vi "SMO.UI.Splash.GetProtectedEvents.vi"(8 "error in (no error)":errorcluster, 11 "SMO.UI.Splash in":refnum<class "SMO.UI.Splash.lvclass">) -> (0 "error out":errorcluster, 2 "Protected Events":T1, 3 "SMO.UI.Splash out":refnum<class "SMO.UI.Splash.lvclass">)   [LabVIEW 2013, in "SMO.UI.Splash.lvclass"]
uses:
  SMO.UI.Splash.lvclass
  Typedefs/ProtectedEvents--Cluster.ctl
  Typedefs/DisplayMessage--Cluster.ctl
  SMO.UI.Splash.lvclass/SMO.UI.Splash.ctl
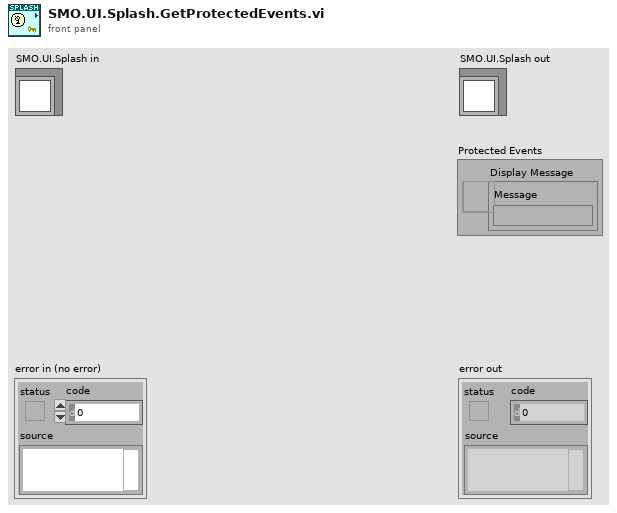
[diagram p1: front panel]
types:
  T1 = typedef "SMO.UI.Splash.lvclass/ProtectedEvents--Cluster.ctl" = cluster{"Display Message":T2}
  T2 = typedef "SMO.UI.Splash.lvclass/DisplayMessage--Cluster.ctl" = refnum<user-event>
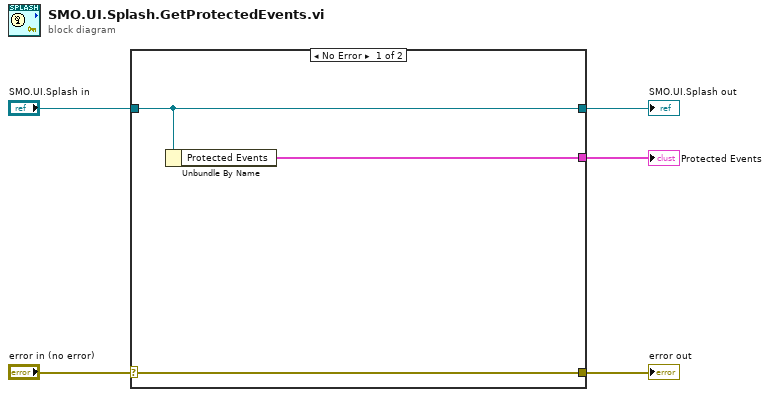
[diagram p0: block diagram]
diagram:
  n1 = case shown="No Error" "error in (no error)" {
    selector: "error in (no error)" -> [w8 w10]
    tunnel: [w8 w10] -> w4
    tunnel: [w7 w9] -> w2
    tunnel: "SMO.UI.Splash in" -> [w7 w9]
    tunnel: [w6 _] -> w1
    frame No Error {
      n2 = Unbundle By Name(w7) -> ("Protected Events"=w6:T1)
    }
    frame Error {
    }
  }
  "error out" <- w4
  "SMO.UI.Splash out" <- w2
  "Protected Events" <- w1
